vi "Calculate_3D_Move_Time.vi"(6 "Model:    Roll        Pitch         Yaw  (deg)":sgl[](array[numeric]), 7 "Work in Tunnel Coordinates":T1, 8 "Backlash?":bool, 9 "Traverse Setup":string, 10 "Positions":sgl[][](array[numeric]), 11 "Start Position":sgl[](array[numeric])) -> (3 "Time (s)":sgl)   [LabVIEW 2022 SP3]
uses:
  DriveConfigGlobal.vi
  Anemometry/Anemometry Sub Vis/Controls/Tunnel_Coordinates.ctl
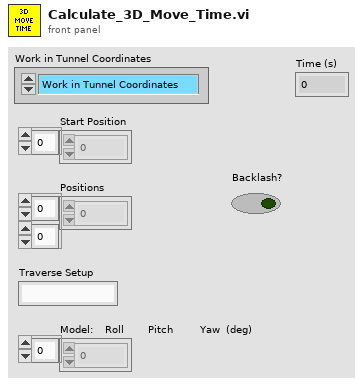
[diagram p1: front panel]
types:
  T1 = typedef "Tunnel_Coordinates.ctl" = enum16{"Work in Tunnel Coordinates", "Work in Model Coordinates"}
  T2 = typedef "DriveProperties.ctl" = cluster{"Channel Name":string, "Vel. Default":sgl, "Acc. Default":sgl, "Vel. Max":sgl, "Vel. Min":sgl, "Acc. Max":sgl, "Acc. Min":sgl, "Pulses/unit":sgl, "Address":u8, "Pulse Offset":i32, "Pos Tolerance":sgl, "Pulses/rev":sgl, "Backlash/Eng units":sgl, "Current Pos":sgl, "Ch Status":enum16{"Active", "Offline", "Simulate"}, "Port Name":string, "Axis Transform mode":string, "Metadata Ch Name":string, "Type":string, "De Power Motor":enum16{"TRUE", "FALSE"}, "ConfigString":string}
  T3 = enum16{"To Traverse Coordinates", "To User Coordinates"}
  T4 = cluster{"Total travel time":sgl, "Accel time":sgl, "Accel fractional distance":sgl}
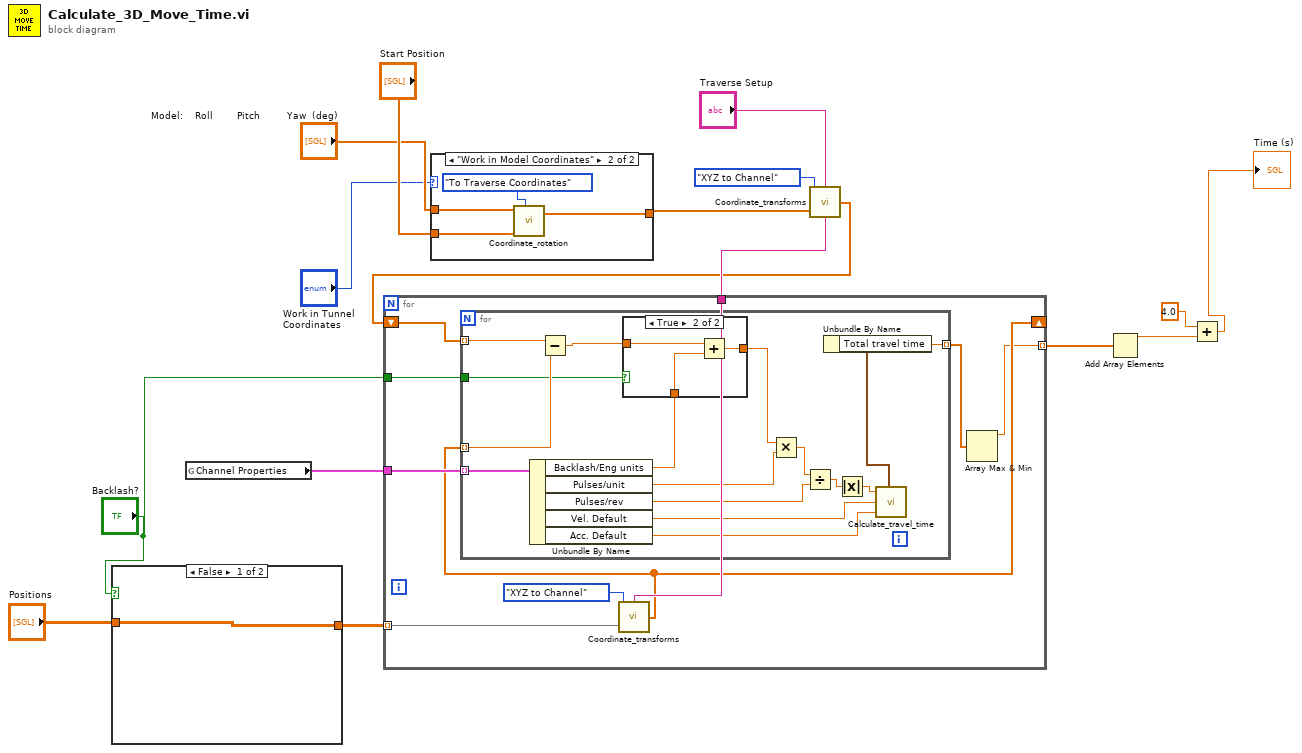
[diagram p0: block diagram]
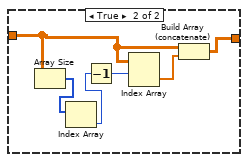
[diagram p2: hidden frame]
diagram:
  n1 = case shown="False" "Backlash?" {
    tunnel: "Positions" -> [w16 w19]
    tunnel: [w16 w17] -> w2
    frame False {
    }
    frame True {
      n2 = Array Size(array=w19) -> (size(s)=w21:i32[])
      n3 = Index Array(array=w21) -> (element=w20:i32)  [unwired: 1 in]
      n4 = Decrement(x=w20) -> (x-1=w22:i32)
      n5 = Index Array(array=w19, index (row)=w22) -> (element=w18:sgl[])  [unwired: 1 in]
      n6 = Build Array (concatenate)(w19, w18) -> (w17:sgl[][])
    }
  }
  n7 = global read "DriveConfigGlobal.vi" "Channel Properties"() -> (w10:T2[])
  n8 = case shown="\"Work in Model Coordinates\"" "Work in Tunnel Coordinates" {
    tunnel: "Start Position" -> [w23 w25]
    tunnel: [w23 w26] -> w7
    tunnel: "Model:    Roll        Pitch         Yaw  (deg)" -> [_ w24]
    frame "Work in Tunnel Coordinates" {
    }
    frame "Work in Model Coordinates" {
      n9 = call "Coordinate_rotation.vi"("Roll-Pitch-Yaw"=w24, "Input Position"=w25, "Mode"=T3."To Traverse Coordinates") -> ("Output Position"=w26:sgl[])  [unwired: 2 in, 1 out]
    }
  }
  n10 = call "Coordinate_transforms.vi"("Traverse Name"="Traverse Setup", "Input"=w7, "Mode"=enum16{"XYZ to Channel", "Channel to XYZ"}."XYZ to Channel") -> ("Output"=w8:sgl[])
  n11 = for {
    shift-right: [w30] -> _
    shift-left: w8 -> [w33]
    tunnel: "Traverse Setup" -> [w35]
    tunnel: w2 -> [w34] mode=indexing
    tunnel: w10 -> [w32]
    tunnel: [w29] -> w11 mode=indexing
    tunnel: "Backlash?" -> [w28]
    n12 = call "Coordinate_transforms.vi"("Traverse Name"=w35, "Input"=w34, "Mode"=enum16{"XYZ to Channel", "Channel to XYZ"}."XYZ to Channel") -> ("Output"=w30:sgl[])
    n13 = for {
      tunnel: w33 -> [w52] mode=indexing
      tunnel: w30 -> [w51] mode=indexing
      tunnel: w32 -> [w50] mode=indexing
      tunnel: [w43] -> w31 mode=indexing
      tunnel: w28 -> [w37]
      n14 = Unbundle By Name(w50) -> ("Backlash/Eng units"=w39:sgl, "Pulses/unit"=w49:sgl, "Pulses/rev"=w47:sgl, "Vel. Default"=w46:sgl, "Acc. Default"=w45:sgl)
      n15 = Subtract(x=w52, y=w51) -> (x-y=w38:sgl)
      n16 = case shown="True" w37 {
        tunnel: [w53 w56] -> w40
        tunnel: w39 -> [_ w55]
        tunnel: w38 -> [w53 w54]
        frame False {
        }
        frame True {
          n17 = Add(x=w54, y=w55) -> (x+y=w56:sgl)
        }
      }
      n18 = Multiply(x=w40, y=w49) -> (x*y=w48:sgl)
      n19 = Divide(x=w48, y=w47) -> (x/y=w42:sgl)
      n20 = Absolute Value(x=w42) -> (abs(x)=w41:sgl)
      n21 = call "Calculate_travel_time.vi"("Default Acceleration Revs/s^2"=w45, "Default Velocity Revs/s"=w46, "Revs to travel"=w41) -> ("Times"=w44:T4)
      n22 = Unbundle By Name(w44) -> ("Total travel time"=w43:sgl)
    }
    n23 = Array Max & Min(array=w31) -> (max value=w29:sgl)  [unwired: 3 out]
  }
  n24 = Add Array Elements(numeric array=w11) -> (sum=w13:sgl)
  n25 = Add(x=sgl 4.0, y=w13) -> (x+y=→"Time (s)":sgl)
